vi "Modtag_Billede-Steffen’s MacBook Pro.vi"() -> ()   [LabVIEW 2018]
uses:
  <vilib>/myRIO/Instrument Drivers/Onboard IO/UART/typedef/VISA Configuration.ctl
  <vilib>/Instr/_visa.llb/VISA Configure Serial Port (Instr).vi
  <vilib>/myRIO/Express VI/Onboard IO/UART/UART Express VI.xnode
  <vilib>/myRIO/Instrument Drivers/Onboard IO/UART/UART.lvlib
panel:
  out "Intensity Graph 4":u8[][](graph)
  in  "Rotation \nOrientation":bool
  out "Array 2":u8[](array[numeric])
  out "Boolean 2":bool
  out "Boolean":bool
  out "Array":u8[](array[numeric])
  out "element":i32
  out "Intensity Graph 7":u8[][](graph)
  out "length":i32
  out "array":u8[](array[numeric])
  out "size(s) 2":i32
  out "Intensity Graph 6":u8[][](graph)
  out "size(s)":i32[](array[numeric])
  out "appended array":u8[][](array[numeric])
  in  "stop":bool
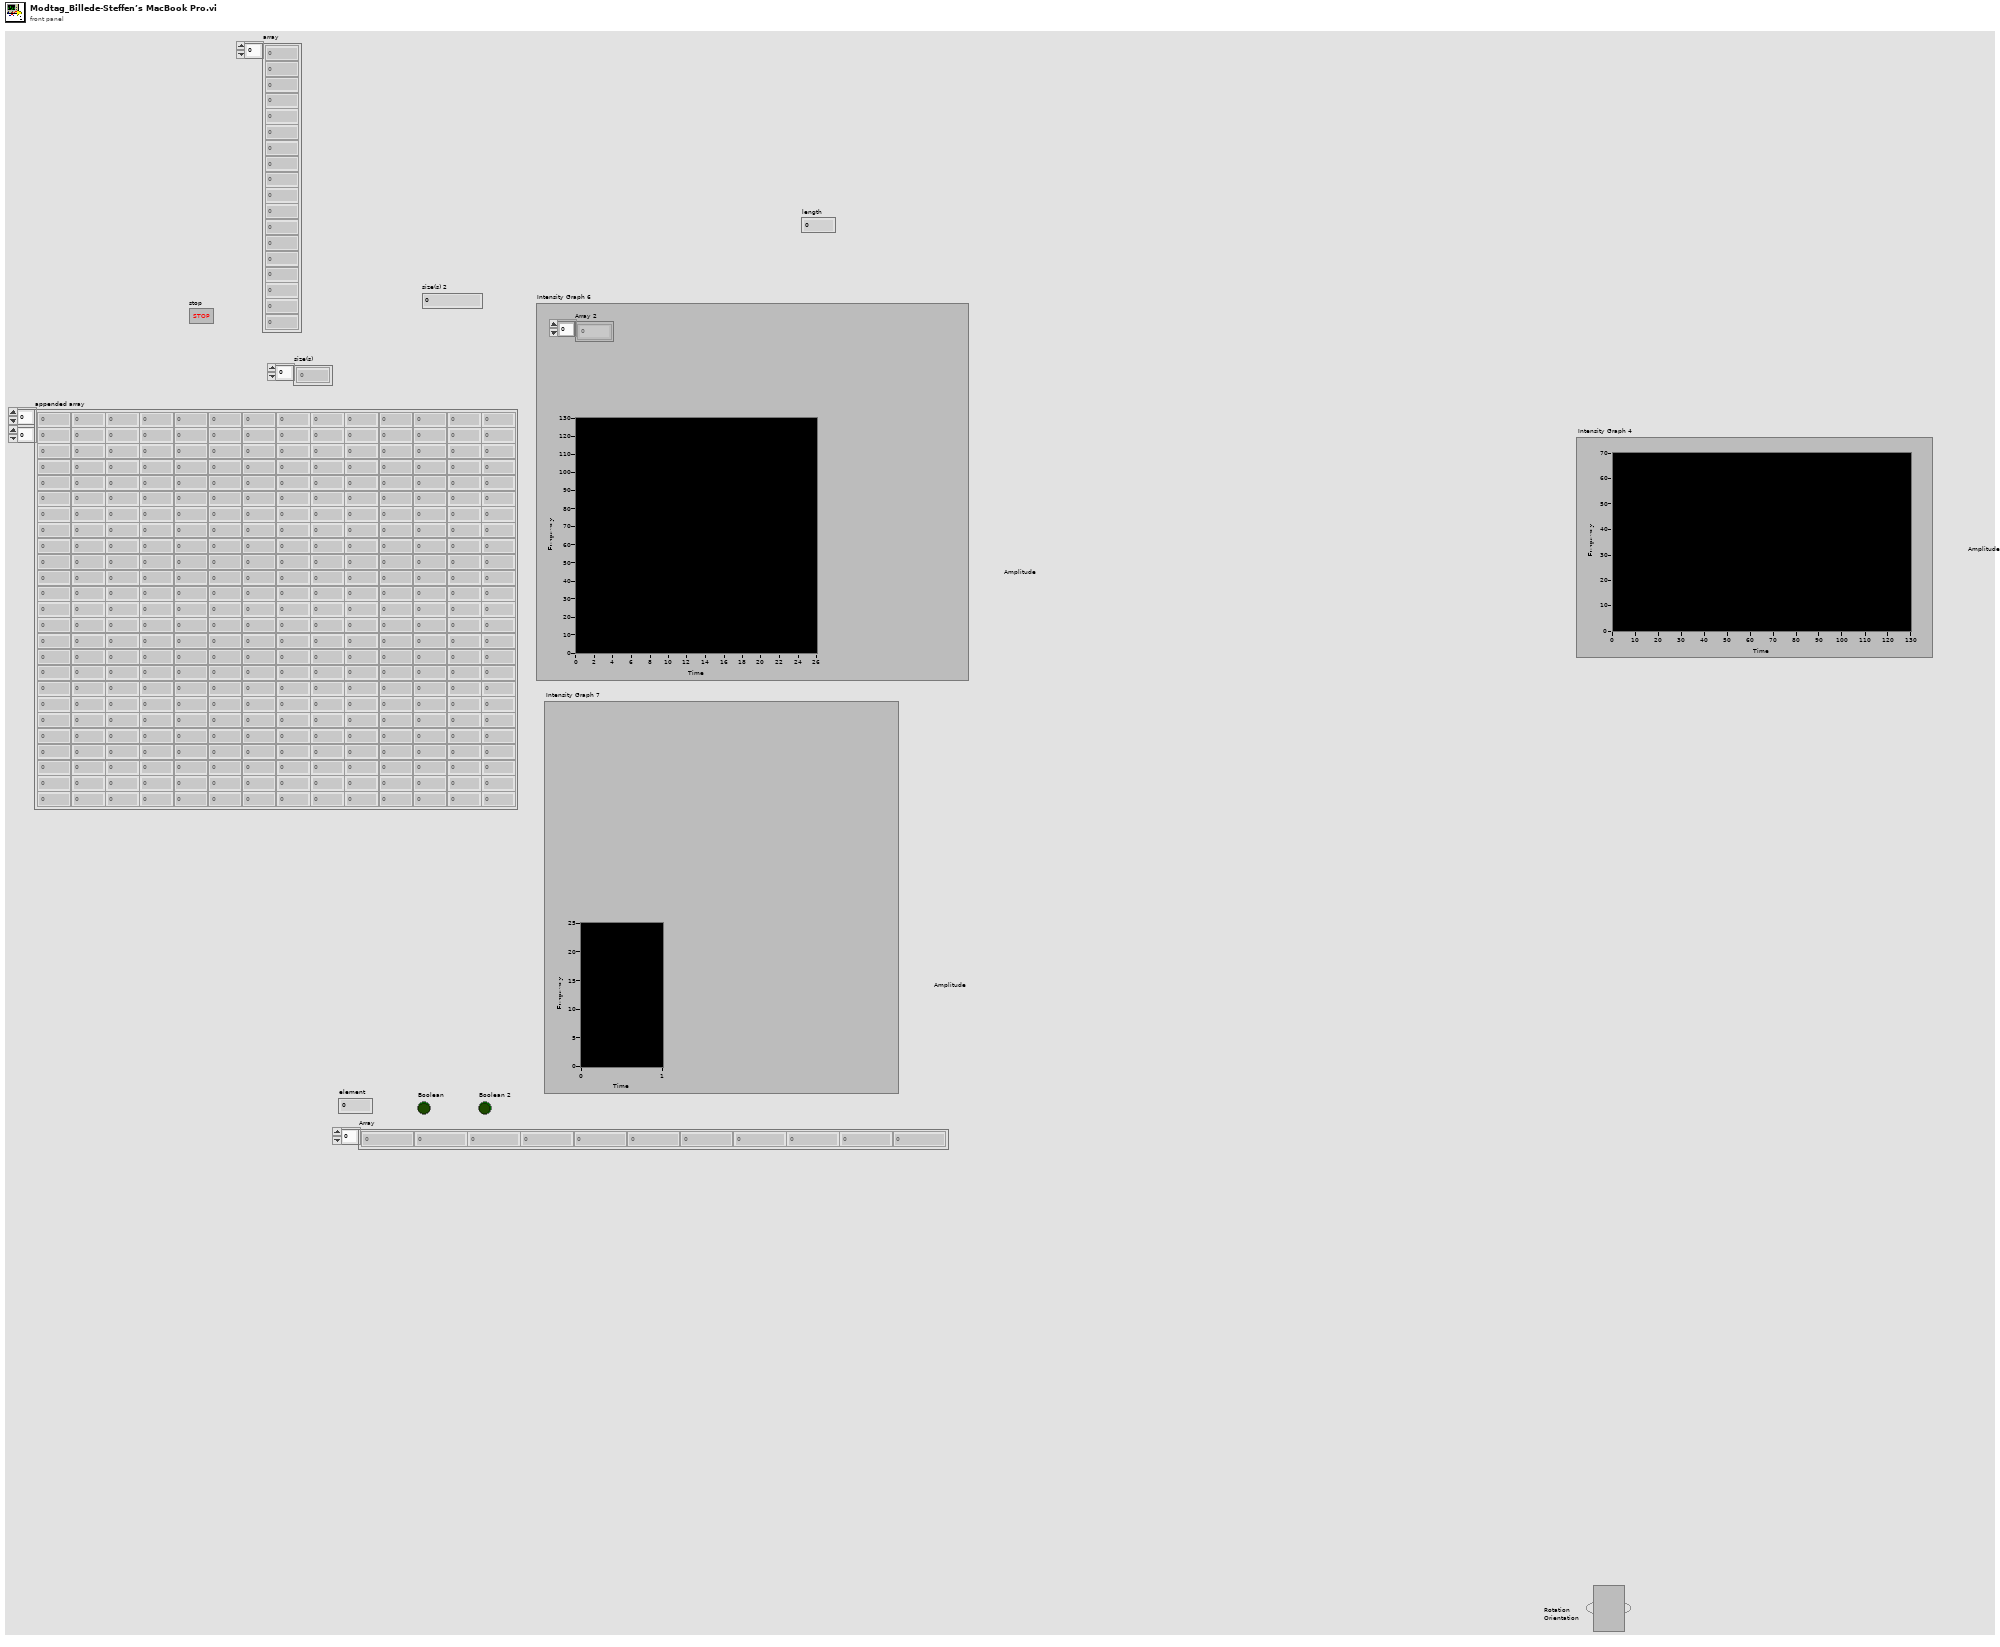
[diagram p1: front panel]
types:
  T1 = typedef "UART.lvlib/VISA Configuration.ctl" = cluster{"baud rate (9600)":u32, "data bits (8)":u16, "parity (0:none)":enum16{"None", "Odd", "Even", "Mark", "Space"}, "stop bits (10: 1 bit)":u16, "flow control (0:none)":u16, "termination char\n(0xA = '\\n' = LF) ":u8, "Enable Termination\nChar (T)":bool, "timeout (10sec)":u32}
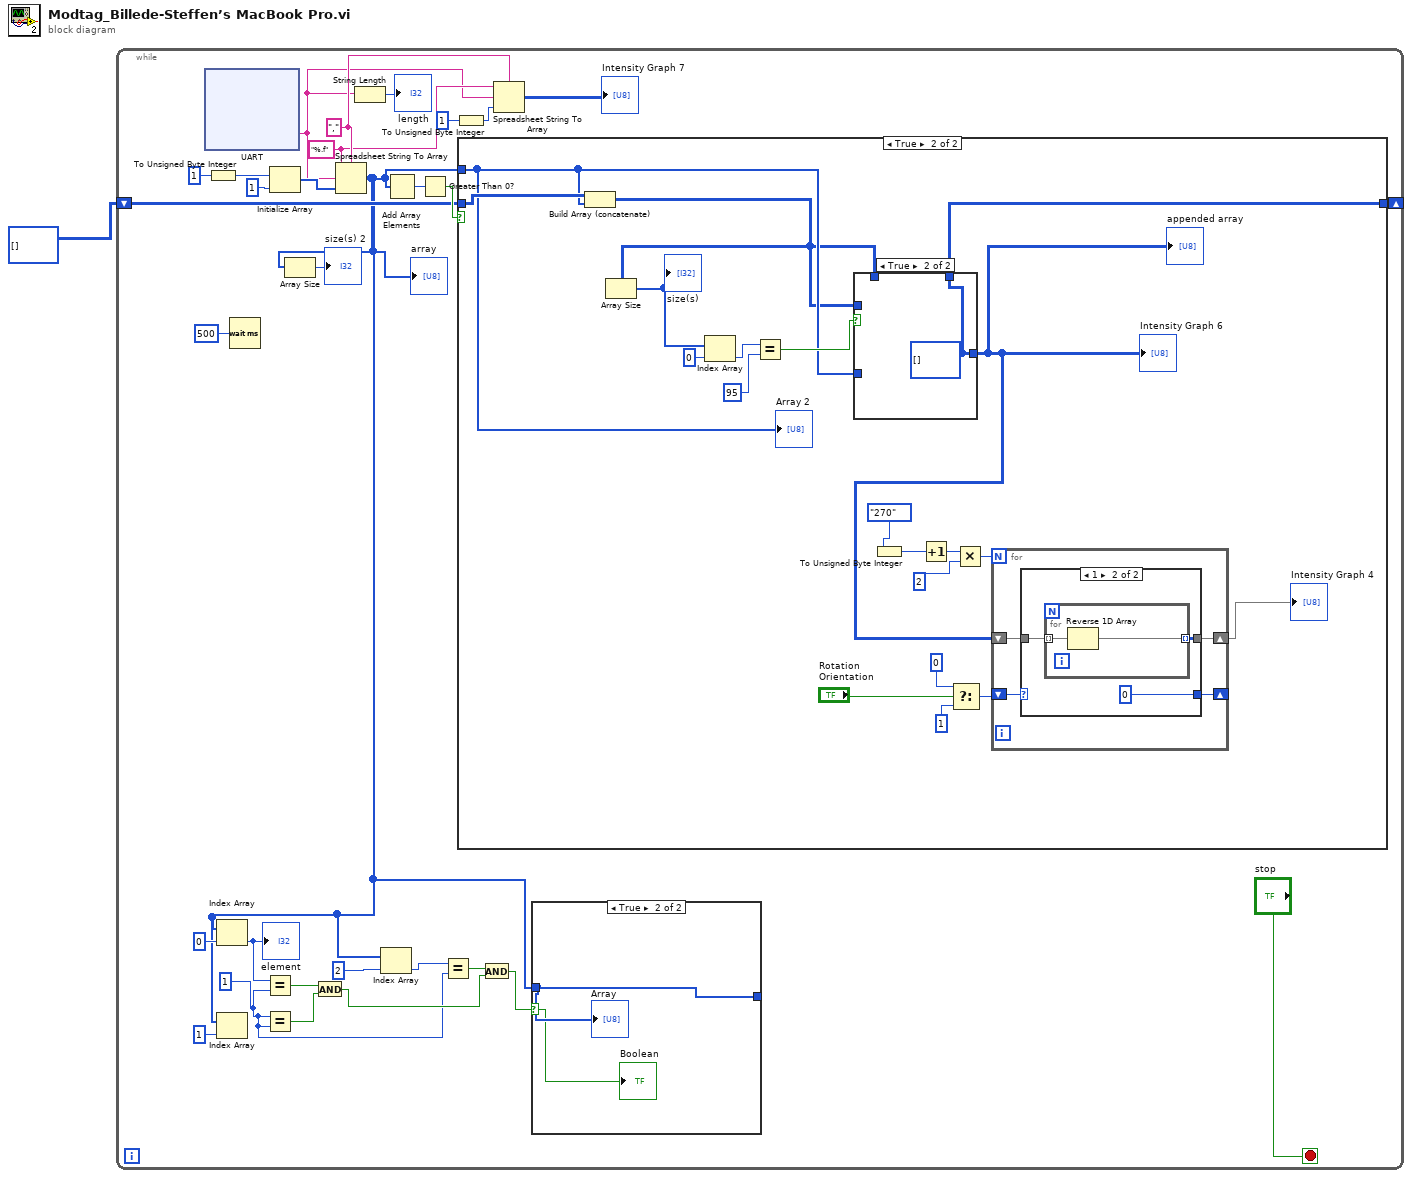
[diagram p0: block diagram]
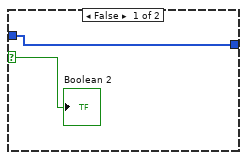
[diagram p2: hidden frame]
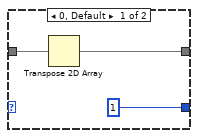
[diagram p4: hidden frame]
diagram:
  n1 = while {
    shift-right: [w25] -> _
    shift-left: u8[][] [] -> [w26]
    stop <- "stop" stop-if-true
    w3 = u8 1 ("y")
    w20 = "," ("delimiter (Tab)")
    w19 = "%.f" ("format string")
    n2 = xnode "UART"() -> ("Characters Read"=w2:string)  [unwired: 1 in, 1 out]
    n3 = To Unsigned Byte Integer(number=u8 1) -> (unsigned 8bit integer=w23:u8)
    n4 = Wait (ms)(milliseconds to wait=u32 500) -> ()  [unwired: 1 out]
    n5 = Equal?(x=w3, y=w3) -> (x = y?=w10:bool)
    n6 = Initialize Array(w23, 1 ("dimension size")) -> (w18:u8[])
    n7 = Spreadsheet String To Array(delimiter (Tab)=w20, format string=w19, spreadsheet string=w2, array type (2D Dbl)=w18) -> (array=w8:u8[])
    "array" <- w8
    n8 = Index Array(array=w8, index=0) -> (element=w13:u8)
    "element" <- w13
    n9 = Index Array(array=w8, index=1) -> ()  [unwired: 1 out]
    n10 = Equal?(x=w13, y=w3) -> (x = y?=w12:bool)
    n11 = Array Size(array=w8) -> (size(s)=→"size(s) 2":i32)
    n12 = And(x=w12, y=w10) -> (x .and. y?=w5:bool)
    n13 = String Length(string=w2) -> (length=→"length":i32)
    n14 = Index Array(array=w8, index=2) -> (element=w7:u8)
    n15 = Add Array Elements(numeric array=w8) -> (sum=w28:u8)
    n16 = Greater Than 0?(x=w28) -> (x > 0?=w27:bool)
    n17 = Equal?(x=w7, y=w3) -> (x = y?=w6:bool)
    n18 = To Unsigned Byte Integer(number=u8 1) -> (unsigned 8bit integer=w15:u8)
    n19 = case shown="True" w27 {
      tunnel: w8 -> [_ w50]
      tunnel: w26 -> [w36 w56]
      tunnel: [w36 w48] -> w25
      frame False {
      }
      frame True {
        n20 = Build Array (concatenate)(w56, w50) -> (w49:u8[][])
        n21 = Array Size(array=w49) -> (size(s)=w55:i32[])
        "size(s)" <- w55
        n22 = Index Array(array=w55, index=0) -> (element=w53:i32)
        n23 = Equal?(x=w53, y=95) -> (x = y?=w51:bool)
        n24 = case shown="True" w51 {
          tunnel: w50 -> [_ _]
          tunnel: w49 -> [w70 _]
          tunnel: [w70 w71] -> w37
          tunnel: w49 -> [w69 _]
          tunnel: [w69 w71] -> w48
          frame False {
          }
          frame True {
            w71 = u8[][] []
          }
        }
        "appended array" <- w37
        "Intensity Graph 6" <- w37
        n25 = To Unsigned Byte Integer(number=enum8{"90", "180", "270"}."270" ("Rotation")) -> (unsigned 8bit integer=w39:u8)
        n26 = Increment(x=w39) -> (x+1=w41:u8)
        n27 = Select(t=u8 0, s="Rotation \nOrientation", f=u8 1) -> (s? t:f=w43:u8)
        n28 = Multiply(x=w41, y=u8 2) -> (x*y=w42:u8)
        n29 = for {
          N: w42 -> [_]
          shift-right: [w59] -> w38
          shift-left: w37 -> [w60]
          shift-right: [w57] -> _
          shift-left: w43 -> [w58]
          n30 = case shown="1" w58 {
            tunnel: w60 -> [w62 w66]
            tunnel: [w63 w65] -> w59
            tunnel: [u8 1 u8 0] -> w57
            frame 0, Default {
              n31 = Transpose 2D Array(2D array=w62) -> (transposed array=w63:u8[][])
            }
            frame 1 {
              n32 = for {
                tunnel: w66 -> [w68] mode=indexing
                tunnel: [w67] -> w65 mode=indexing
                n33 = Reverse 1D Array(array=w68) -> (reversed array=w67:u8[])
              }
            }
          }
        }
        "Intensity Graph 4" <- w38
        "Array 2" <- w50
      }
    }
    n34 = And(x=w6, y=w5) -> (x .and. y?=w4:bool)
    n35 = Spreadsheet String To Array(delimiter (Tab)=w20, format string=w19, spreadsheet string=w2, array type (2D Dbl)=w15) -> (array=→"Intensity Graph 7":u8[][])
    n36 = case shown="True" w4 {
      selector: w4 -> [w32 w34]
      tunnel: w8 -> [w33 w35]
      tunnel: [w33 w35] -> _
      frame False {
        "Boolean 2" <- w32
      }
      frame True {
        "Array" <- w35
        "Boolean" <- w34
      }
    }
  }
